vi "test2.vi"() -> ()   [LabVIEW 2014]
uses:
  <vilib>/Utility/file.llb/Write To Spreadsheet File (DBL).vi
panel:
  out "Action":i64
  in  "Save":bool
  in  "Stop":bool
  in  "Start":bool
  in  "Time Delay in Sec":dbl=1.0
  out "XY Graph":cluster{"Y":dbl[], "Y":dbl[]}[](graph)=[{"Y"=[0.0, 6.0, 7.0, 8.0, 9.0, 10.0], "Y"=[0.0, 0.4506452001265784, 0.8342457747634698, 0.030796541605822902, 0.11721293885320039, 0.8396632251315854]}]
  in  "stop":bool
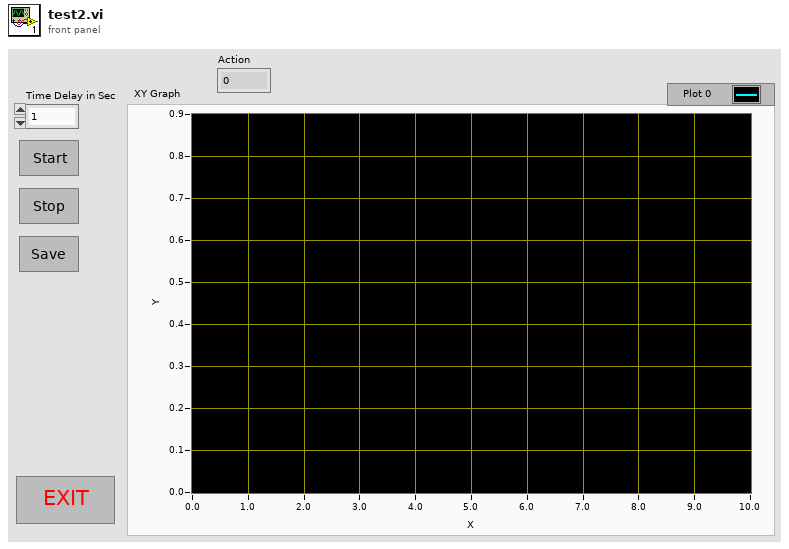
[diagram p1: front panel]
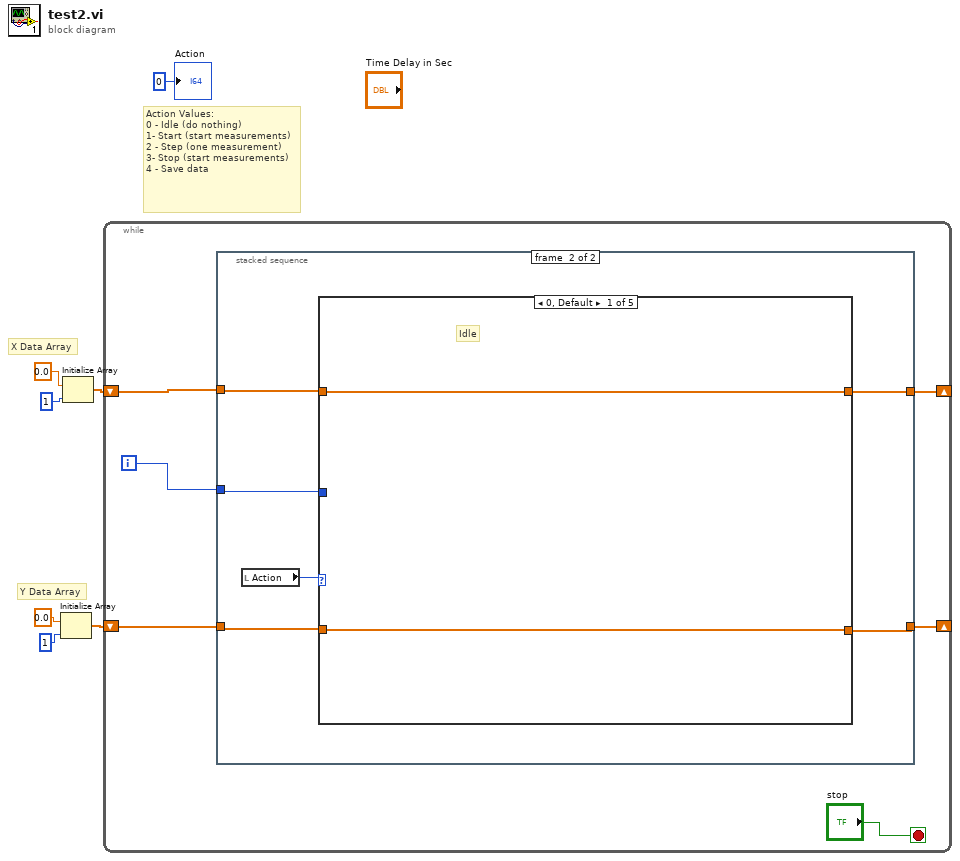
[diagram p0: block diagram]
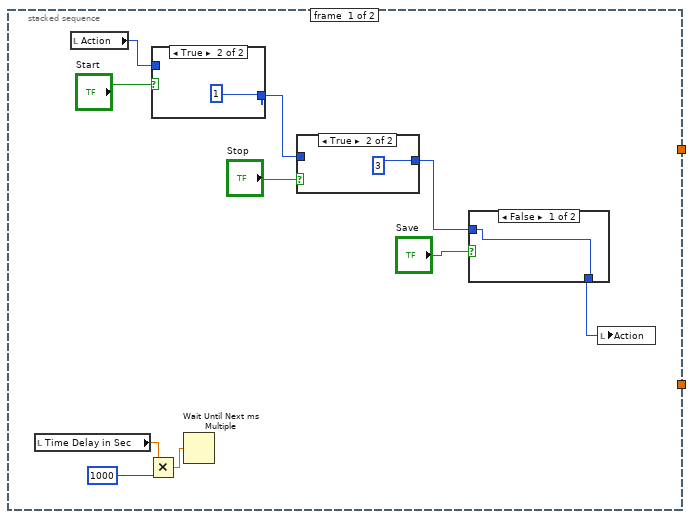
[diagram p2: hidden frame]
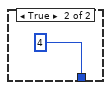
[diagram p3: hidden frame]
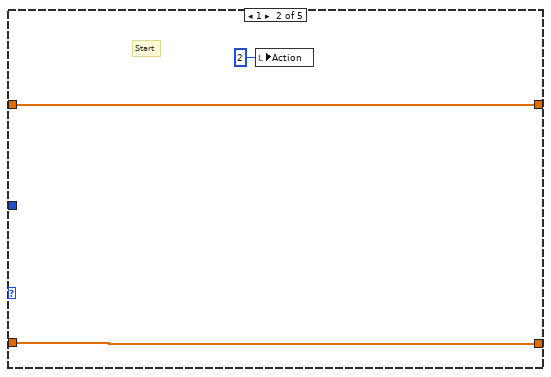
[diagram p6: hidden frame]
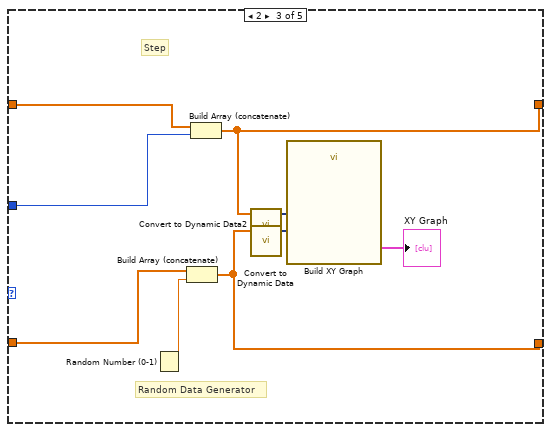
[diagram p7: hidden frame]
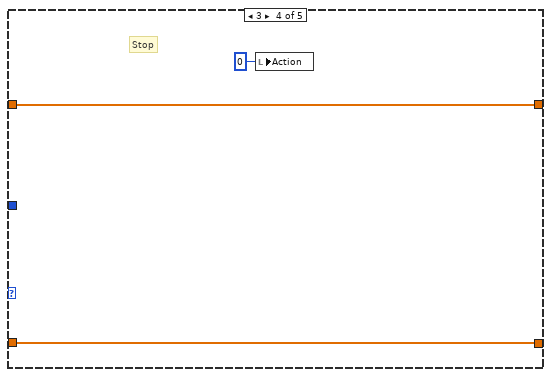
[diagram p8: hidden frame]
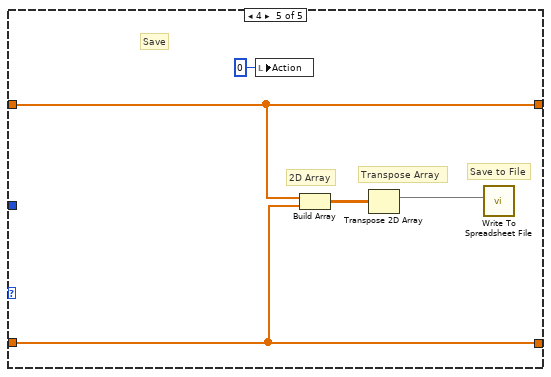
[diagram p9: hidden frame]
diagram:
  # "Y Data Array"
  # "X Data Array"
  # "Action Values:\n0 - Idle (do nothing)\n1- Start (start measurements)\n2 - Step (one measurement)\n3- Stop (start measurements)\n4 - Save data"
  n1 = Initialize Array(0.0 ("element"), 1 ("dimension size")) -> (w2:dbl[])
  n2 = Initialize Array(0.0 ("element"), 1 ("dimension size")) -> (w6:dbl[])
  n3 = while {
    shift-right: [w9] -> _
    shift-left: w6 -> [w12]
    shift-right: [w10] -> _
    shift-left: w2 -> [w11]
    i -> [w8]
    stop <- "stop" stop-if-true
    n4 = stacked-sequence {
      tunnel: w12 -> [_ w35]
      tunnel: w11 -> [_ w34]
      tunnel: [_ w33] -> w10
      tunnel: [_ w32] -> w9
      tunnel: w8 -> [_ w31]
      frame #0 {
        n5 = local read "Time Delay in Sec"() -> (w17:dbl)
        n6 = local read "Action"() -> (w14:i64)
        n7 = Multiply(x=w17, y=u32 1000 ("millisecond multiple")) -> (x*y=w16:dbl)
        n8 = case shown="True" "Start" {
          tunnel: w14 -> [w28 _]
          tunnel: [w28 1] -> w20
          frame False {
          }
          frame True {
          }
        }
        n9 = Wait Until Next ms Multiple(millisecond multiple=w16) -> ()  [unwired: 1 out]
        n10 = case shown="True" "Stop" {
          tunnel: w20 -> [w26 _]
          tunnel: [w26 3] -> w19
          frame False {
          }
          frame True {
          }
        }
        n11 = case shown="False" "Save" {
          tunnel: w19 -> [w24 _]
          tunnel: [w24 4] -> w15
          frame False {
          }
          frame True {
          }
        }
        n12 = local write "Action"(w15) -> ()
      }
      frame #1 {
        n13 = local read "Action"() -> (w30:i64)
        n14 = case shown="0, Default" w30 {
          tunnel: w35 -> [w37 w39 w48 w52 w56]
          tunnel: w34 -> [w36 w38 w47 w51 w55]
          tunnel: [w36 w38 w45 w51 w55] -> w33
          tunnel: [w37 w39 w43 w52 w56] -> w32
          tunnel: w31 -> [_ _ w41 _ _]
          frame 0, Default {
            # "Idle"
          }
          frame 1 {
            # "Start"
            n15 = local write "Action"(i64 2 ("Action")) -> ()
          }
          frame 2 {
            # "Step"
            # "Random Data Generator"
            n16 = Random Number (0-1)() -> (number: 0 to 1=w46:dbl)
            n17 = Build Array (concatenate)(w47, w46) -> (w45:dbl[])
            n18 = Build Array (concatenate)(w48, w41) -> (w43:dbl[])
            n19 = call "Convert to Dynamic Data2"("Array"=w43) -> ("Dynamic Data Type"=w42:dynamicdata)  [unwired: 3 in]
            n20 = call "Convert to Dynamic Data"("Array"=w45) -> ("Dynamic Data Type"=w44:dynamicdata)  [unwired: 3 in]
            n21 = call "Build XY Graph"("Y Input"=w44, "X Input"=w42) -> ("XY Graph"=→"XY Graph":cluster{"X":dbl[], "Y":dbl[]}[])  [unwired: 8 in, 1 out]
          }
          frame 3 {
            # "Stop"
            n22 = local write "Action"(i64 0 ("Action")) -> ()
          }
          frame 4 {
            # "Transpose Array"
            # "Save to File"
            # "2D Array"
            # "Save"
            n23 = local write "Action"(i64 0 ("Action")) -> ()
            n24 = Build Array(w56, w55) -> (w54:dbl[][])
            n25 = Transpose 2D Array(2D array=w54) -> (transposed array=w53:dbl[][])
            n26 = call-poly <vilib>:"Write To Spreadsheet File.vi"("2D data"=w53) -> ()  [unwired: 7 in, 1 out]
          }
        }
      }
    }
  }
  "Action" <- i64 0 ("Action")
